vi "estacion_terrena.vi"() -> ()   [LabVIEW 2023]
uses:
  <vilib>/Instr/_visa.llb/VISA Configure Serial Port (Instr).vi
  <vilib>/picture/3D Picture Control/NI_3D Picture Control.lvlib
panel:
  in  "baud rate (9600)":u32=9600
  out "String 7":string="7:32:58 PM"
  out "String 6":string="7/26/2023"
  out "Ace1":i32(graph)
  out "Ace3":i32(graph)
  out "Ace2":i32(graph)
  out "Z":string="1"
  out "Altura":dbl(slide)=28.854625550660792 scale=0.0..50.0
  out "Y":string="-4.5"
  out "X":string="2.3"
  out "Longitud":string="-99.43"
  out "Latitud":string="19.99"
  out "Humedad":dbl=78.13953488372093 format="%#_4g"
  out "XY Graph 3":cluster{dbl[], dbl[]}[](graph) caption="XY Graph"
  out "Temperatura":dbl=28.0 format="%#_4g"
  out "Presión":dbl=78.13953488372093 format="%#_4g"
  out "XY Graph 2":cluster{dbl[], dbl[]}[](graph) caption="XY Graph"
  in  "Blank Button":bool
  out "XY Graph":cluster{dbl[], dbl[]}[](graph)
  out "read buffer":string
  in  "COM":refnum<visa-resource-name>
  out "3D Picture":refnum<vi>(3d-picture)
  # "ALTITUD"
  # "HUMEDAD RELATIVA"
  # "m"
  # "%"
  # "PRESSURE"
  # "GPS"
  # "LATITUD"
  # "hPa"
  # "LONGITUD"
  # "TEMPERATURA\nINTERNA"
  # "X"
  # "Y"
  # "°C"
  # "Z"
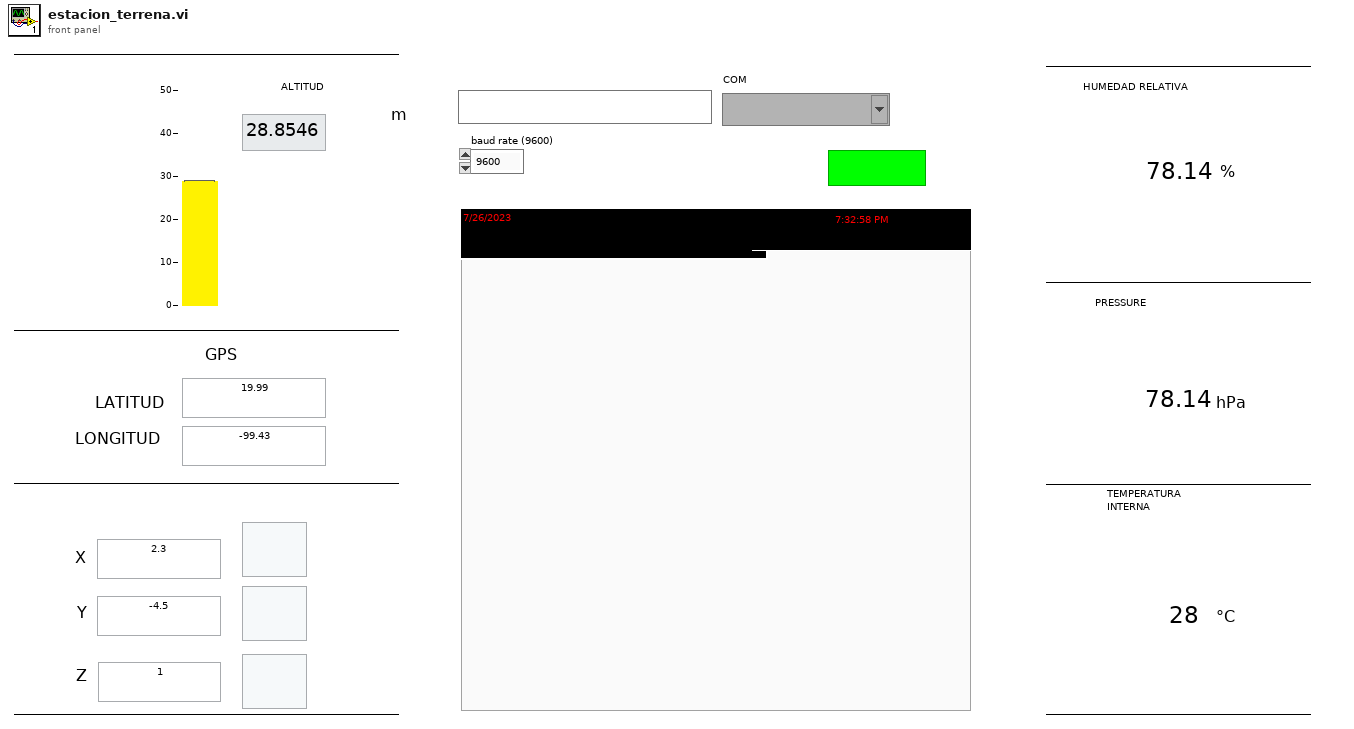
[diagram p1: front panel]
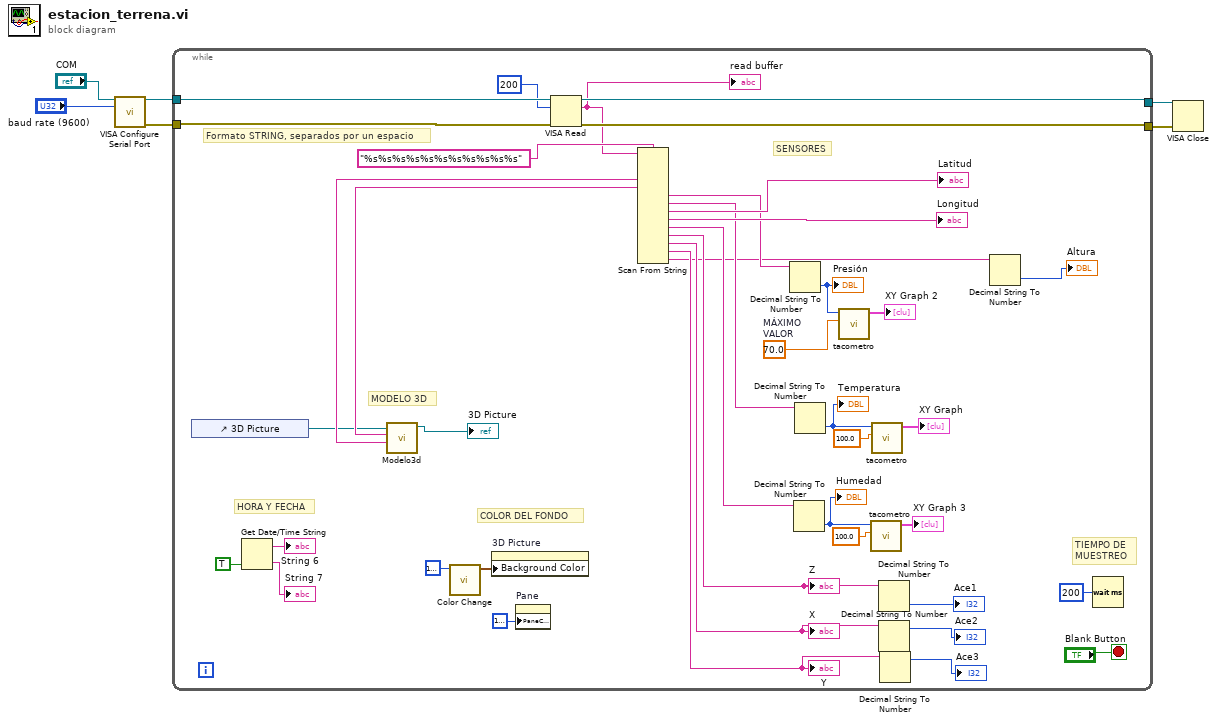
[diagram p0: block diagram]
diagram:
  n1 = call-poly "VISA Configure Serial Port"("VISA resource name"="COM", "baud rate (9600)"="baud rate (9600)") -> ("VISA resource name out"=w5:refnum<visa-resource-name>, "error out"=w3:errorcluster)  [unwired: 12 in]
  n2 = while {
    tunnel: w5 -> [w47]
    tunnel: [w46] -> w4
    tunnel: w3 -> [w45]
    tunnel: [w44] -> w2
    stop <- "Blank Button" stop-if-true
    w37 = 70.0  # MÁXIMO  VALOR
    # "TIEMPO DE \nMUESTREO"
    # "SENSORES"
    # "COLOR DEL FONDO"
    # "HORA Y FECHA"
    # "MODELO 3D"
    # "Formato STRING, separados por un espacio"
    n3 = control-ref of="3D Picture"() -> (w23:refnum<vi>)
    n4 = Get Date/Time String(want seconds? (F)=TRUE) -> (date string=→"String 6":string, time string=→"String 7":string)  [unwired: 2 in]
    n5 = call <vilib>:"Color Change.vi"("Color"=u32 16777216) -> ("RGBA"=w34:cluster{"R":sgl, "G":sgl, "B":sgl, "A":sgl})  [unwired: 10 in]
    n6 = property on="3D Picture" class="SceneGraphDisp (strict)"("Background Color"=w34) -> ()  [unwired: 2 in, 2 out]
    n7 = property on="Pane" class="Pane"("PaneColor"=u32 16777226 ("Pane Color")) -> ()  [unwired: 2 in, 2 out]
    n8 = VISA Read(VISA resource name=w47, byte count=u32 200, error in (no error)=w45) -> (VISA resource name out=w46:refnum<visa-resource-name>, read buffer=w7:string, error out=w44:errorcluster)  [unwired: 1 out]
    "read buffer" <- w7
    n9 = Scan From String(format string="%s%s%s%s%s%s%s%s%s%s%s", input string=w7) -> (output 1=w25:string, output 2=w24:string, output 3=w21:string, output 4=w17:string, output 5=→"Latitud":string, output 6=→"Longitud":string, output 7=w16:string, output 8=w15:string, output 9=w14:string, output 10=w13:string, output 11=w12:string)  [unwired: 13 in, 3 out]
    "X" <- w14
    "Y" <- w13
    "Z" <- w15
    n10 = call "Modelo3d.vi"("String 2"=w25, "String"=w24, "SceneGraphDisplay in"=w23) -> ("SceneNode out"=→"3D Picture":refnum<vi>)  [unwired: 8 in]
    n11 = Decimal String To Number(string=w21) -> (number=w20:i32)  [unwired: 2 in, 1 out]
    "Presión" <- w20
    n12 = Decimal String To Number(string=w16) -> (number=w18:i32)  [unwired: 2 in, 1 out]
    "Humedad" <- w18
    n13 = Decimal String To Number(string=w17) -> (number=w19:i32)  [unwired: 2 in, 1 out]
    "Temperatura" <- w19
    n14 = call "tacometro.vi"("MÁXIMO \nVALOR"=w37, "VALOR\nACTUAL"=w20) -> ("XY Graph"=→"XY Graph 2":cluster{dbl[], dbl[]}[])  [unwired: 9 in]
    n15 = call "tacometro.vi"("MÁXIMO \nVALOR"=100.0 ("MÁXIMO \nVALOR"), "VALOR\nACTUAL"=w18) -> ("XY Graph"=→"XY Graph 3":cluster{dbl[], dbl[]}[])  [unwired: 9 in]
    n16 = call "tacometro.vi"("MÁXIMO \nVALOR"=100.0 ("MÁXIMO \nVALOR"), "VALOR\nACTUAL"=w19) -> ("XY Graph"=→"XY Graph":cluster{dbl[], dbl[]}[])  [unwired: 9 in]
    n17 = Decimal String To Number(string=w15) -> (number=→"Ace1":i32)  [unwired: 2 in, 1 out]
    n18 = Decimal String To Number(string=w14) -> (offset past number=→"Ace2":i32)  [unwired: 2 in, 1 out]
    n19 = Decimal String To Number(string=w13) -> (offset past number=→"Ace3":i32)  [unwired: 2 in, 1 out]
    n20 = Decimal String To Number(string=w12) -> (number=→"Altura":i32)  [unwired: 2 in, 1 out]
    n21 = Wait (ms)(milliseconds to wait=u32 200) -> ()  [unwired: 1 out]
  }
  n22 = VISA Close(VISA resource name=w4, error in (no error)=w2) -> ()  [unwired: 1 out]
